vi "C4LV_releaseAllInterfaces.vi"(0 "c4if Arr in":refnum<k24>[](array[refnum]), 11 "error in (no error)":errorcluster) -> (15 "error out":errorcluster)   [LabVIEW 2015, in "libC4HdlLV.lvlib"]
uses:
  libC4HdlLV.lvlib
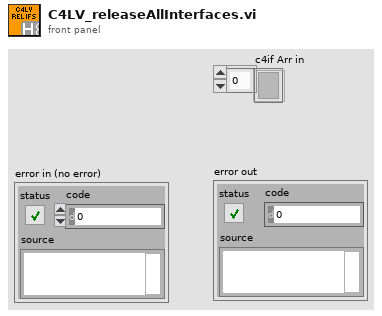
[diagram p1: front panel]
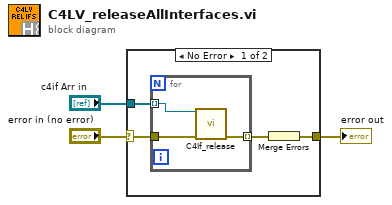
[diagram p0: block diagram]
diagram:
  n1 = case shown="No Error" "error in (no error)" {
    selector: "error in (no error)" -> [w4 w11]
    tunnel: "c4if Arr in" -> [w7 _]
    tunnel: [w5 w11] -> w3
    frame No Error {
      n2 = for {
        tunnel: w7 -> [w8] mode=indexing
        tunnel: w4 -> [w10]
        tunnel: [w9] -> w6 mode=indexing
        n3 = call "C4If_release.vi"("c4if in"=w8, "error in (no error)"=w10) -> ("error out"=w9:errorcluster)  [unwired: 13 in]
      }
      n4 = Merge Errors(w6) -> (w5:errorcluster)
    }
    frame Error {
    }
  }
  "error out" <- w3
